vi "runSingleDPScript.vi"(6 "HWLoop?":bool, 8 "error in (no error)":errorcluster, 9 "index":i32, 10 "status in":refnum<vi>, 11 "ExperimentRunner in":refnum<class "ExperimentRunner.lvclass">) -> (0 "error out":errorcluster, 2 "status out":refnum<vi>, 3 "ExperimentRunner out":refnum<class "ExperimentRunner.lvclass">)   [LabVIEW 2011, in "Views.lvlib" / "ExperimentControl.lvlib" / "ExperimentRunner.lvclass"]
doc: "Run a single script"
uses:
  ExperimentRunner.lvclass
  ExperimentRunner.lvclass/ExperimentRunner.ctl
  Hal/HWController/HWControllerEvents/HWControllerEvents.lvclass
  Tools/Filing/FileNeologist/FileNeologist.lvclass
  Tools/Filing.lvlib
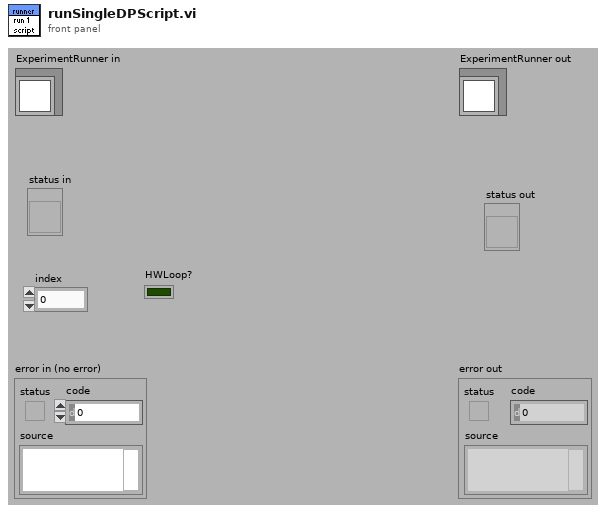
[diagram p1: front panel]
types:
  T1 = enum16{"Ready", "Compiling", "Configured", "Running", "Stopping", "Unresolved Error"}
  T2 = enum16{"start", "stop", "statusInquiry", "configure", "resetError", "resourcesInquiry", "reserveResources", "initialise", "resetAllChannels", "staticUpdate", "close", "HWStatus", "error", "resourcesAvailable", "resourcesReserved"}
  T3 = cluster{"incomingEventTypes":cluster{"start":cluster{"Boolean":bool}, "stop":cluster{"Boolean":bool}, "statusInquiry":cluster{"Boolean":bool}, "configure":cluster{"DPScriptPath":path, "TimeStamp":string, "HWLoop?":bool}, "resetError":cluster{"Boolean":bool}, "resourcesInquiry":cluster{"Boolean":bool}, "reserveResources":cluster{"HWList":string[]}, "initialise":cluster{"HWList":string[]}, "close":cluster{"Boolean":bool}, "resetAllChannels":cluster{"Boolean":bool}, "staticChannelUpdate":cluster{"channel_address":string, "calibratedValue":dbl}, "runScript":cluster{"DPScriptPath":path, "TimeStamp":string, "HWLoop?":bool}, "compilingScript":cluster{"Path":path}, "compiledScript":cluster{"Path":path, "timeCompileAt":string}, "compilerError":cluster{"Path":path}, "configureCompiledScript":cluster{"DPScriptPath":path, "TimeStamp":string, "HWLoop?":bool, "CompiledScript":cluster{"ScriptListCompiler.lvclass":refnum<class "ScriptListCompiler.lvclass">, "aoChannels":refnum<class "AnalogOutput.lvclass">[], "doChannels":refnum<class "DigitalOutput.lvclass">[], "rfChannels":refnum<class "DDSOutput.lvclass">[]}}, "restartCompiler":cluster{"restart":bool}, "staticRfChannelUpdate":cluster{"channel_address":string, "Output":cluster{"Frequency(MHz)":dbl, "Amplitude":dbl, "Phase":dbl, "OutputForm":enum16{"Sine", "Square", "Triangle", "Arbitrary"}}}, "cameraUpdate":cluster{"Camera":string, "Type":string, "settings":path}}, "outgoingEventTypes":cluster{"HWStatus":cluster{"status":enum16{"Ready", "Compiling", "Configured", "Running", "Stopping", "Unresolved Error"}}, "error":cluster{"error out":errorcluster}, "resourcesAvailable":cluster{"availableHWList":string[], "reservedHWList":string[]}, "resourcesReserved":cluster{"reservedHWList":string[]}}}
  T4 = cluster{"DPScriptPath":path, "TimeStamp":string, "HWLoop?":bool}
  T5 = cluster{"eventId":enum16{"start", "stop", "statusInquiry", "configure", "resetError", "resourcesInquiry", "reserveResources", "initialise", "resetAllChannels", "staticUpdate", "close", "HWStatus", "error", "resourcesAvailable", "resourcesReserved"}, "configure":cluster{"DPScriptPath":path, "TimeStamp":string, "HWLoop?":bool}}
  T6 = cluster{"eventId":enum16{"start", "stop", "statusInquiry", "configure", "resetError", "resourcesInquiry", "reserveResources", "initialise", "resetAllChannels", "staticUpdate", "close", "HWStatus", "error", "resourcesAvailable", "resourcesReserved"}, "start":cluster{"Boolean":bool}}
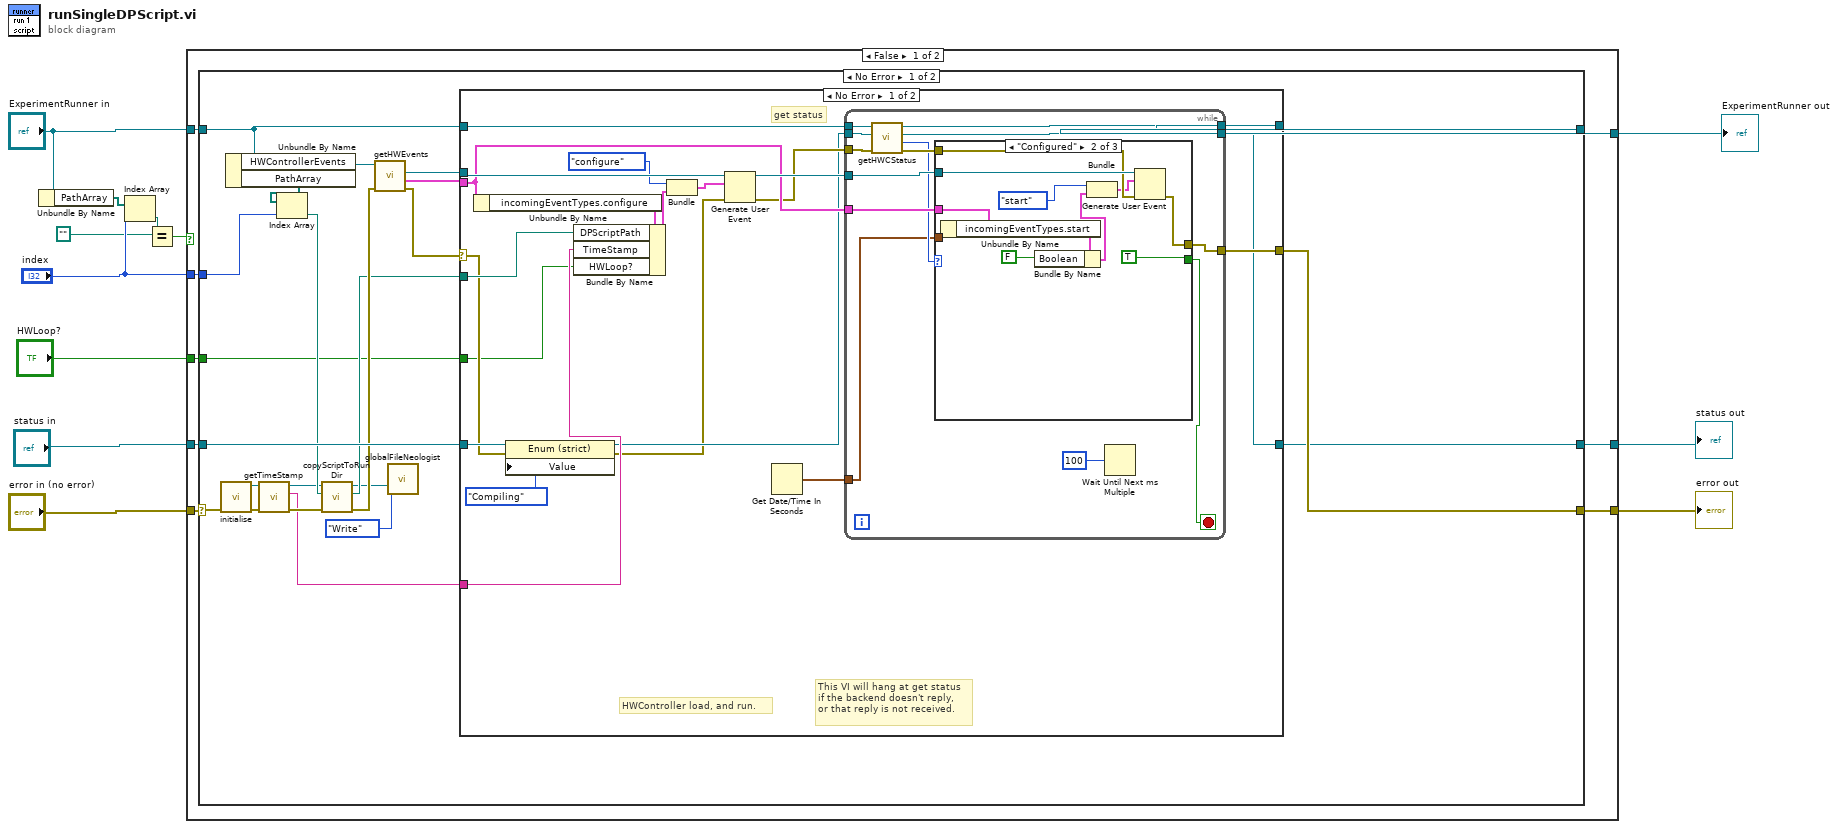
[diagram p0: block diagram]
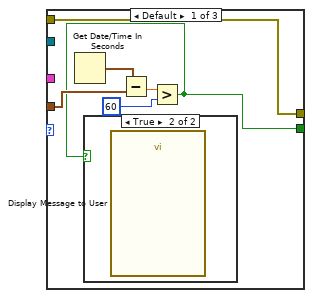
[diagram p2: hidden frame]
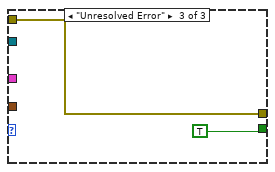
[diagram p4: hidden frame]
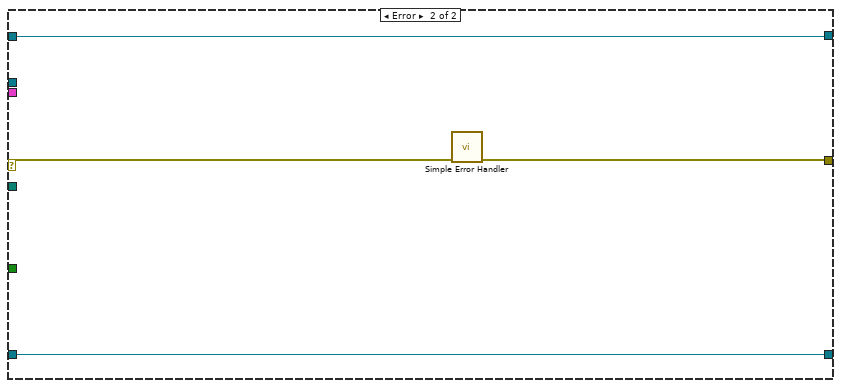
[diagram p5: hidden frame]
diagram:
  n1 = Unbundle By Name("ExperimentRunner in") -> ("PathArray"=w7:path[])
  n2 = Index Array(array=w7, index="index") -> (element=w5:path)
  n3 = Equal?(x=w5, y=path "") -> (x = y?=w3:bool)
  n4 = case shown="False" w3 {
    tunnel: "error in (no error)" -> [w20 w103]
    tunnel: [w19 w103] -> w11
    tunnel: [w18 w105] -> w10
    tunnel: "status in" -> [w17 w104]
    tunnel: [w16 w104] -> w9
    tunnel: "ExperimentRunner in" -> [w15 w105]
    tunnel: "index" -> [w14 _]
    tunnel: "HWLoop?" -> [w13 _]
    frame False {
      n5 = case shown="No Error" w20 {
        selector: w20 -> [w32 w102]
        tunnel: [w41 w102] -> w19
        tunnel: [w25 w101] -> w18
        tunnel: w15 -> [w37 w101]
        tunnel: w14 -> [w42 _]
        tunnel: w17 -> [w36 w100]
        tunnel: [w35 w100] -> w16
        tunnel: w13 -> [w21 _]
        frame No Error {
          n6 = call "initialise.vi"("error in (no error)"=w32) -> ("error out"=w31:errorcluster, "FileNeologist out"=w30:refnum<class "FileNeologist.lvclass">)  [unwired: 9 in]
          n7 = Unbundle By Name(w37) -> ("HWControllerEvents"=w40:refnum<class "HWControllerEvents.lvclass">, "PathArray"=w43:path[])
          n8 = call "getTimeStamp.vi"("error in (no error)"=w31, "FileNeologist in"=w30) -> ("error out"=w28:errorcluster, "TimeStamp"=w26:string, "FileNeologist out"=w27:refnum<class "FileNeologist.lvclass">)  [unwired: 7 in]
          n9 = Index Array(array=w43, index=w42) -> (element=w29:path)
          n10 = call-dynamic "copyScriptToRunDir.vi"("error in (no error)"=w28, "Path in"=w29, "FileNeologist in"=w27) -> ("error out"=w34:errorcluster, "Path out"=w33:path, "FileNeologist out"=w24:refnum<class "FileNeologist.lvclass">)  [unwired: 6 in]
          n11 = call-dynamic "getHWEvents.vi"("error in (no error)"=w34, "HWControllerEvents in"=w40) -> ("error out"=w22:errorcluster, "eventDataTypes"=w38:T3, "HWCEvent"=w39:refnum<user-event>)  [unwired: 6 in, 1 out]
          n12 = call "globalFileNeologist.vi"("FileNeologist in"=w24, "Action"=enum16{"Write", "Read"}."Write") -> ()  [unwired: 9 in, 1 out]
          n13 = case shown="No Error" w22 {
            selector: w22 -> [w45 w99]
            tunnel: [w57 w98] -> w41
            tunnel: w39 -> [w64 _]
            tunnel: w38 -> [w58 _]
            tunnel: w33 -> [w62 _]
            tunnel: w37 -> [w52 w97]
            tunnel: [w53 w97] -> w25
            tunnel: w36 -> [w49 w96]
            tunnel: [w51 w96] -> w35
            tunnel: w26 -> [w56 _]
            tunnel: w21 -> [w44 _]
            frame No Error {
              # "This VI will hang at get status\nif the backend doesn't reply,\nor that reply is not received."
              # "get status"
              # "HWController load, and run."
              n14 = Unbundle By Name(w58) -> ("incomingEventTypes.configure"=w63:T4)
              n15 = property class="Enum (strict)"(reference=w49, error in=w45, "Value"=T1."Compiling") -> (reference out=w48:refnum<vi>, error out=w46:errorcluster)
              n16 = Bundle By Name(cluster=w63, "DPScriptPath"=w62, "TimeStamp"=w56, "HWLoop?"=w44) -> (w61:T4)
              n17 = Bundle("eventId"=T2."configure", "configure"=w61) -> (w60:T5)  [unwired: 1 in]
              n18 = Generate User Event(user event=w64, event data cluster=w60, error in=w46) -> (user event out=w59:refnum<user-event>, error out=w54:errorcluster)
              n19 = Get Date/Time In Seconds() -> (seconds since 1Jan1904=w50:timestamp)
              n20 = while {
                tunnel: w59 -> [w77]
                tunnel: w58 -> [w76]
                tunnel: [w75] -> w57
                tunnel: w54 -> [w74]
                tunnel: [w72] -> w53
                tunnel: w52 -> [w71]
                tunnel: w48 -> [w70]
                tunnel: [w69] -> w51
                tunnel: w50 -> [w66]
                stop <- w65 stop-if-true
                n21 = call "getHWCStatus.vi"("error in (no error)"=w74, "status in"=w70, "ExperimentRunner in"=w71) -> ("error out"=w73:errorcluster, "status"=w68:T1, "status out"=w69:refnum<vi>, "ExperimentRunner out"=w72:refnum<class "ExperimentRunner.lvclass">)  [unwired: 5 in]
                n22 = case shown="\"Configured\"" w68 {
                  tunnel: w77 -> [_ w93 _]
                  tunnel: w76 -> [_ w92 _]
                  tunnel: [w83 w91 w94] -> w75
                  tunnel: w73 -> [w83 w90 w94]
                  tunnel: [w78 TRUE TRUE] -> w65
                  tunnel: w66 -> [w81 _ _]
                  frame Default {
                    n23 = Get Date/Time In Seconds() -> (seconds since 1Jan1904=w82:timestamp)
                    n24 = Subtract(x=w82, y=w81) -> (x-y=w80:dbl)
                    n25 = Greater?(x=w80, y=60) -> (0:w78:bool)
                    n26 = case shown="True" w78 {
                      frame False {
                      }
                      frame True {
                        n27 = call "Display Message to User"() -> ()  [unwired: 10 in, 2 out]
                      }
                    }
                  }
                  frame "Configured" {
                    n28 = Unbundle By Name(w92) -> ("incomingEventTypes.start"=w88:cluster{"Boolean":bool})
                    n29 = Bundle By Name(cluster=w88, "Boolean"=FALSE) -> (w87:cluster{"Boolean":bool})
                    n30 = Bundle("eventId"=T2."start", "start"=w87) -> (w89:T6)  [unwired: 1 in]
                    n31 = Generate User Event(user event=w93, event data cluster=w89, error in=w90) -> (error out=w91:errorcluster)  [unwired: 1 out]
                  }
                  frame "Unresolved Error" {
                  }
                }
                n32 = Wait Until Next ms Multiple(millisecond multiple=100) -> ()  [unwired: 1 out]
              }
            }
            frame Error {
              n33 = call <vilib>:"Simple Error Handler.vi"("error in (no error)"=w99) -> ("error out"=w98:errorcluster)  [unwired: 4 in, 4 out]
            }
          }
        }
        frame Error {
        }
      }
    }
    frame True {
    }
  }
  "error out" <- w11
  "ExperimentRunner out" <- w10
  "status out" <- w9
